vi "LidarTest_VMX.vi"() -> ()   [LabVIEW 2019]
uses:
  Z:/Git/LV2020/builds/StudicaLidarForVMX/VMX/StudicaLidar_VMX Lvlibp/StudicaLidar_VMX.lvlibp
panel:
  out "angle":sgl
  out "min dis":sgl
  out "distance 2":sgl
  out "max value":sgl
  out "min value":sgl
  out "distance":sgl
  out "Lidar dt":u32
  out "XY Graph":cluster{sgl[], sgl[]}(graph)
  out "Angle(degree)/Point":sgl[](array[numeric])
  out "Distance(mm)/Point":sgl[](array[numeric])
  in  "stop":bool
  out "Lidar error":errorcluster
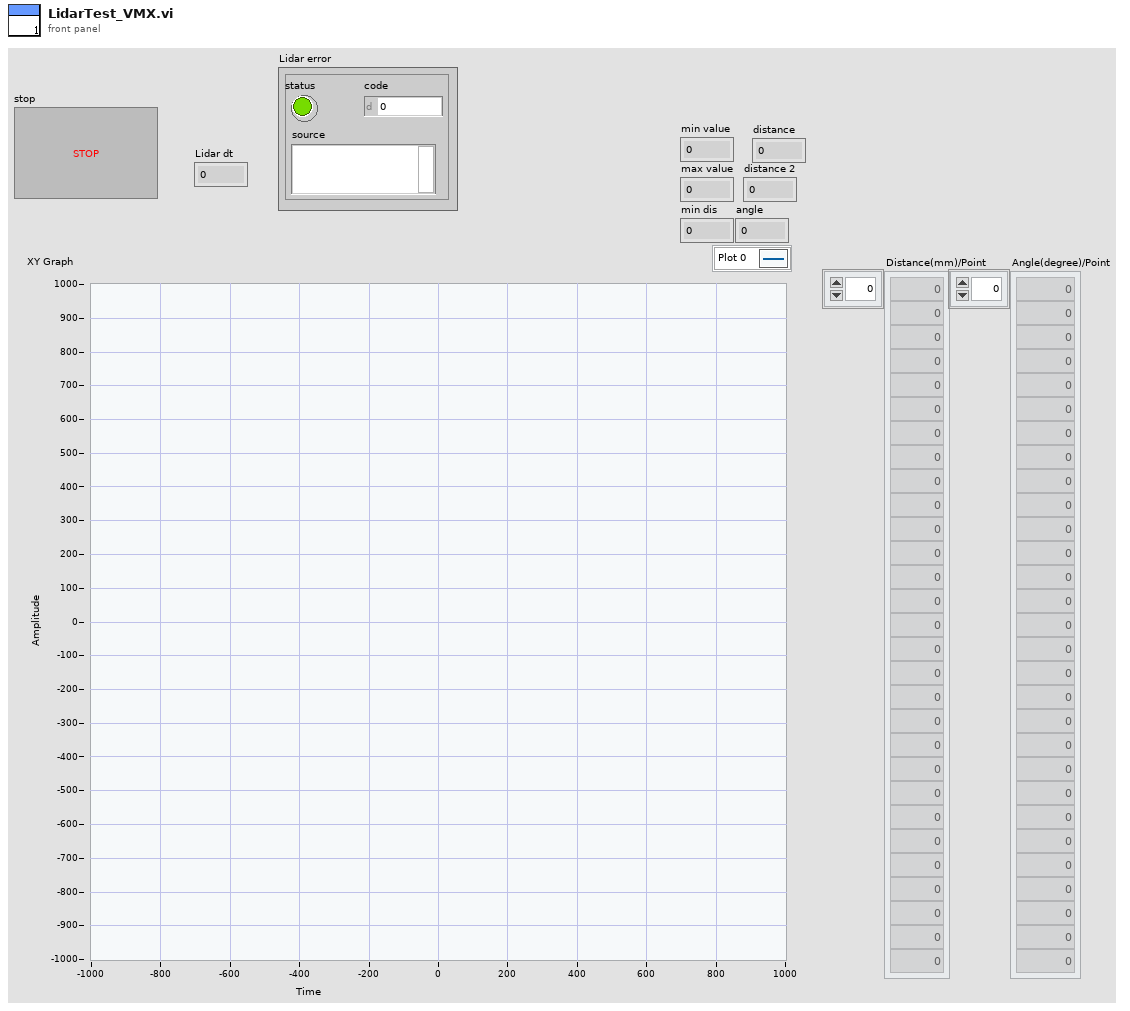
[diagram p1: front panel]
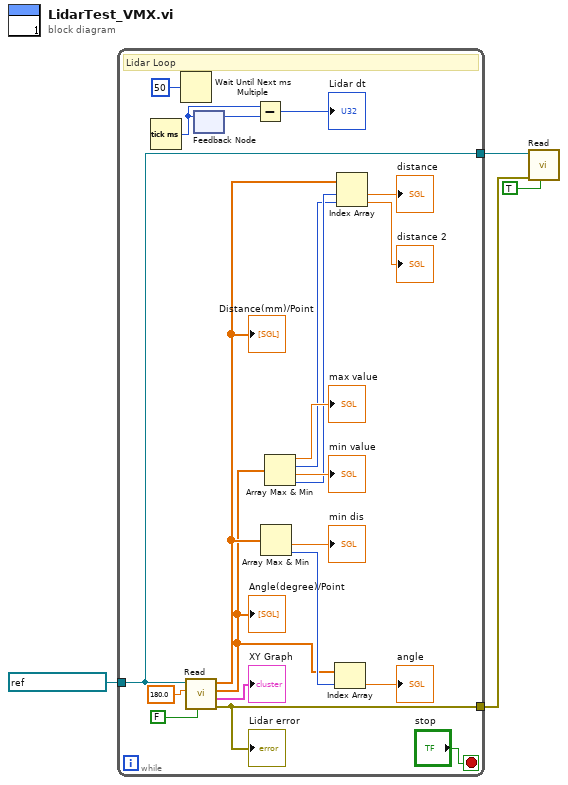
[diagram p0: block diagram]
diagram:
  n1 = while {
    tunnel: refnum<visa-resource-name> "ASRL3::INSTR" ("Select Port") -> [w24]
    tunnel: [w7] -> w3
    tunnel: [w24] -> w1
    stop <- "stop" stop-if-true
    # "Lidar Loop"
    n2 = Tick Count (ms)() -> (millisecond timer value=w20:u32)
    n3 = Wait Until Next ms Multiple(millisecond multiple=u32 50) -> ()  [unwired: 1 out]
    n4 = call "Read.vi"("Clear&Close"=FALSE, "deg diff"=sgl 180.0, "reference"=w24) -> ("error out"=w7:errorcluster, "XY Graph"=→"XY Graph":cluster{sgl[], sgl[]}, "Angle(degree)/Point"=w10:sgl[], "Distance(mm)/Point"=w13:sgl[])  [unwired: 4 in, 1 out]
    "Distance(mm)/Point" <- w13
    "Angle(degree)/Point" <- w10
    "Lidar error" <- w7
    n5 = feedback #1() -> (w21:u32)  [unwired: 1 in]
    n6 = feedback-in #1(w20) -> ()
    n7 = Subtract(x=w20, y=w21) -> (x-y=→"Lidar dt":u32)
    n8 = Array Max & Min(array=w13) -> (min value=→"min dis":sgl, min index (indices)=w11:i32)  [unwired: 2 out]
    n9 = Array Max & Min(array=w10) -> (max value=→"max value":sgl, max index (indices)=w14:i32, min value=→"min value":sgl, min index (indices)=w15:i32)
    n10 = Index Array(array=w10, index=w11) -> (element=→"angle":sgl)
    n11 = Index Array(array=w13, index #1=w15, index #2=w14) -> (element #1=→"distance":sgl, element #2=→"distance 2":sgl)
  }
  n12 = call "Read.vi"("Clear&Close"=TRUE, "error in (no error)"=w3, "reference"=w1) -> ()  [unwired: 4 in, 5 out]
